vi "Core.vi"(8 "Mirrors& Splitters":map{cluster{i32, i32}, string}(c390), 9 "ySize":i32, 10 "xSize":i32, 11 "Initial Lazer":T1) -> (3 "Number Energized":i32)   [LabVIEW 2023, in "d16.lvlib"]
uses:
  d16.lvlib
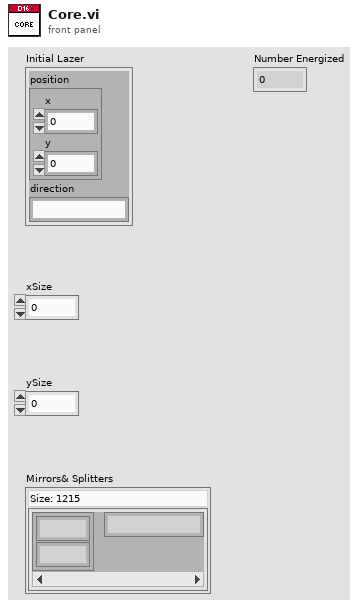
[diagram p1: front panel]
types:
  T1 = cluster{"position":cluster{"x":i32, "y":i32}, "direction":string}
  T2 = set{cluster{"position":cluster{"x":i32, "y":i32}, "direction":string}}
  T3 = cluster{"position":cluster{"x":i32, "y":i32}, "direction":string}[]
  T4 = cluster{"position":cluster{"x":i32, "y":i32}, string}
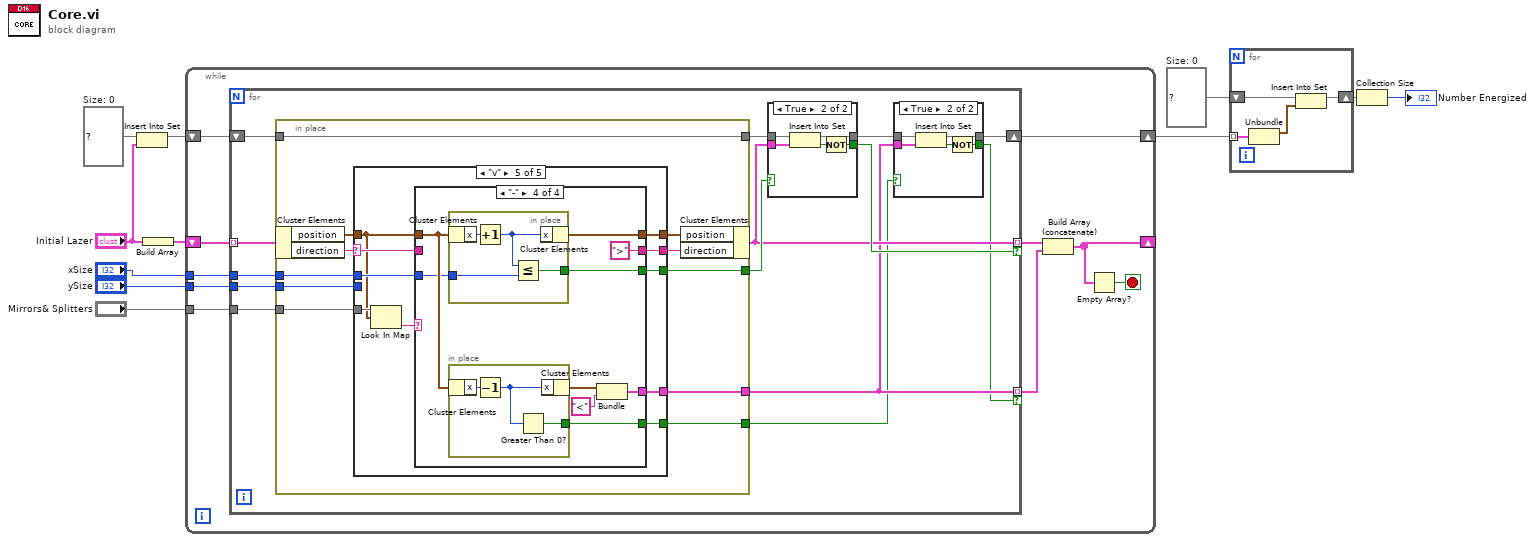
[diagram p0: block diagram]
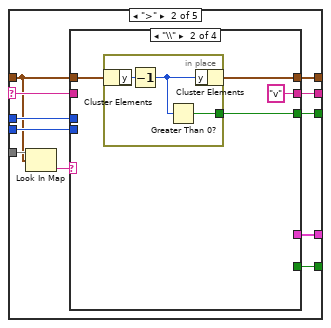
[diagram p5: hidden frame]
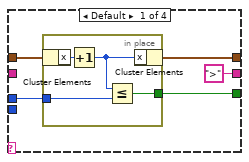
[diagram p6: hidden frame]
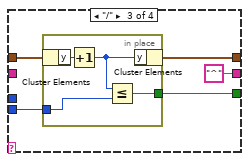
[diagram p7: hidden frame]
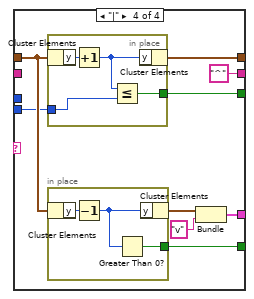
[diagram p8: hidden frame]
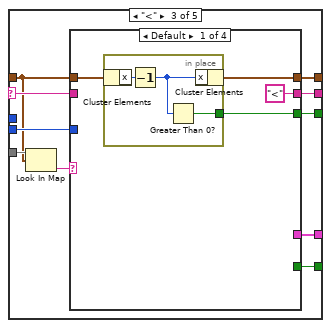
[diagram p9: hidden frame]
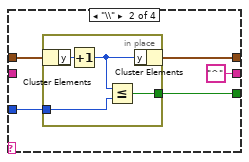
[diagram p10: hidden frame]
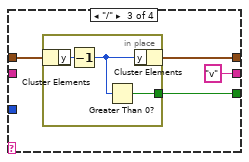
[diagram p11: hidden frame]
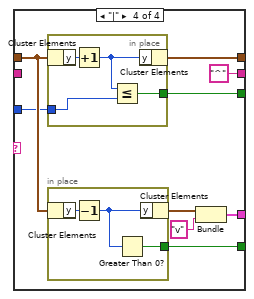
[diagram p12: hidden frame]
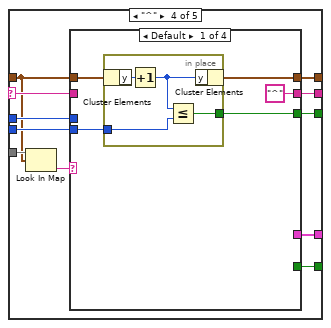
[diagram p13: hidden frame]
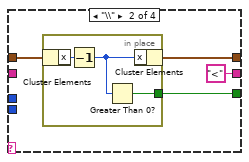
[diagram p14: hidden frame]
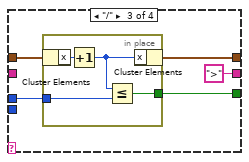
[diagram p15: hidden frame]
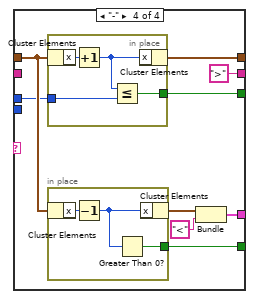
[diagram p16: hidden frame]
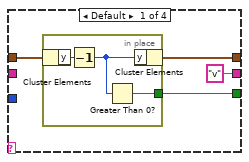
[diagram p17: hidden frame]
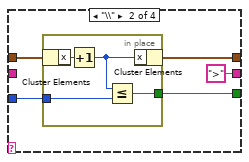
[diagram p18: hidden frame]
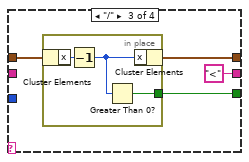
[diagram p19: hidden frame]
diagram:
  w10 = set{cluster{i32, i32}} {}  # Size: 0
  w6 = T2 {}  # Size: 0
  n1 = Insert Into Set(10:"Initial Lazer", 11:w6) -> (3:w7:T2)  [unwired: 1 out]
  n2 = Build Array("Initial Lazer") -> (w5:T3)
  n3 = while {
    tunnel: "xSize" -> [w17]
    tunnel: "ySize" -> [w14]
    shift-right: [w13] -> _
    shift-left: w5 -> [w19]
    tunnel: "Mirrors& Splitters" -> [w18]
    shift-right: [w20] -> w9
    shift-left: w7 -> [w21]
    stop <- w15 stop-if-true
    n4 = for {
      tunnel: w19 -> [w32] mode=indexing
      tunnel: w18 -> [w34]
      tunnel: w17 -> [w33]
      tunnel: [w27] -> w16 mode=indexing if=w28
      tunnel: w14 -> [w31]
      tunnel: [w24] -> w12 mode=indexing if=w22
      shift-right: [w25] -> w20
      shift-left: w21 -> [w35]
      n5 = in-place {
        in-place-border: w35 -> [w58]
        in-place-border: [w58] -> w30
        in-place-border: w34 -> [w57]
        in-place-border: w33 -> [w56]
        in-place-border: [w55] -> w29
        in-place-border: w31 -> [w50]
        in-place-border: [w49] -> w24
        in-place-border: [w48] -> w23
        n6 = in-place-cluster #1(w32) -> ("position"=w54:cluster{"x":i32, "y":i32}, "direction"=w51:string)
        n7 = case shown="\"v\"" w51 {
          selector: w51 -> [_ w65 w116 w166 w217]
          tunnel: w54 -> [w59 w60 w112 w161 w213]
          tunnel: w57 -> [_ w70 w121 w171 w222]
          tunnel: w56 -> [_ w64 _ w165 w216]
          tunnel: [_ w62 w114 w163 w214] -> w55
          tunnel: [_ w68 w119 w169 w220] -> w52
          tunnel: [w59 w63 w115 w164 w215] -> w53
          tunnel: w50 -> [_ w61 w113 w162 _]
          tunnel: [_ w67 w118 w168 w219] -> w48
          tunnel: [_ w66 w117 w167 w218] -> w49
          frame "False", Default {
          }
          frame ">" {
            n8 = Look In Map(map=w70, key=w60) -> (value=w69:string)  [unwired: 1 in, 1 out]
            n9 = case shown="\"\\\\\"" w69 {
              tunnel: [">" "v" "^" "^"] -> w68
              tunnel: [_ _ _ w96] -> w67
              tunnel: [_ _ _ w102] -> w66
              tunnel: w65 -> [_ _ _ _]
              tunnel: w60 -> [w75 w82 w90 w99]
              tunnel: w64 -> [w73 _ _ _]
              tunnel: [w74 w81 w89 w100] -> w63
              tunnel: [w72 w80 w87 w101] -> w62
              tunnel: w61 -> [_ _ w88 w98]
              frame Default {
                n10 = in-place {
                  in-place-border: [w78] -> w72
                  in-place-border: w73 -> [w76]
                  n11 = in-place-cluster #2(w75) -> ("x"=w79:i32)
                  n12 = Increment(x=w79) -> (x+1=w77:i32)
                  n13 = Less Or Equal?(x=w77, y=w76) -> (x <= y?=w78:bool)
                  n14 = in-place-cluster #2("x"=w77) -> (w74:cluster{"x":i32, "y":i32})
                }
              }
              frame "\\" {
                n15 = in-place {
                  in-place-border: [w85] -> w80
                  n16 = in-place-cluster #3(w82) -> ("y"=w86:i32)
                  n17 = Decrement(x=w86) -> (x-1=w84:i32)
                  n18 = Greater Than 0?(x=w84) -> (x > 0?=w85:bool)
                  n19 = in-place-cluster #3("y"=w84) -> (w81:cluster{"x":i32, "y":i32})
                }
              }
              frame "/" {
                n20 = in-place {
                  in-place-border: [w94] -> w87
                  in-place-border: w88 -> [w92]
                  n21 = in-place-cluster #4(w90) -> ("y"=w95:i32)
                  n22 = Increment(x=w95) -> (x+1=w93:i32)
                  n23 = Less Or Equal?(x=w93, y=w92) -> (x <= y?=w94:bool)
                  n24 = in-place-cluster #4("y"=w93) -> (w89:cluster{"x":i32, "y":i32})
                }
              }
              frame "|" {
                n25 = in-place {
                  in-place-border: [w107] -> w101
                  in-place-border: w98 -> [w105]
                  n26 = in-place-cluster #5(w99) -> ("y"=w108:i32)
                  n27 = Increment(x=w108) -> (x+1=w106:i32)
                  n28 = Less Or Equal?(x=w106, y=w105) -> (x <= y?=w107:bool)
                  n29 = in-place-cluster #5("y"=w106) -> (w100:cluster{"x":i32, "y":i32})
                }
                n30 = in-place {
                  in-place-border: [w109] -> w96
                  n31 = in-place-cluster #6(w99) -> ("y"=w111:i32)
                  n32 = Decrement(x=w111) -> (x-1=w110:i32)
                  n33 = Greater Than 0?(x=w110) -> (x > 0?=w109:bool)
                  n34 = in-place-cluster #6("y"=w110) -> (w104:cluster{"x":i32, "y":i32})
                }
                n35 = Bundle("position"=w104, "v") -> (w102:T4)  [unwired: 1 in]
              }
            }
          }
          frame "<" {
            n36 = Look In Map(map=w121, key=w112) -> (value=w120:string)  [unwired: 1 in, 1 out]
            n37 = case shown="Default" w120 {
              tunnel: ["<" "^" "v" "^"] -> w119
              tunnel: [_ _ _ w145] -> w118
              tunnel: [_ _ _ w151] -> w117
              tunnel: w116 -> [_ _ _ _]
              tunnel: w112 -> [w125 w132 w140 w148]
              tunnel: [w124 w131 w139 w149] -> w115
              tunnel: [w123 w130 w138 w150] -> w114
              tunnel: w113 -> [_ w129 _ w147]
              frame Default {
                n38 = in-place {
                  in-place-border: [w127] -> w123
                  n39 = in-place-cluster #7(w125) -> ("x"=w128:i32)
                  n40 = Decrement(x=w128) -> (x-1=w126:i32)
                  n41 = Greater Than 0?(x=w126) -> (x > 0?=w127:bool)
                  n42 = in-place-cluster #7("x"=w126) -> (w124:cluster{"x":i32, "y":i32})
                }
              }
              frame "\\" {
                n43 = in-place {
                  in-place-border: [w136] -> w130
                  in-place-border: w129 -> [w134]
                  n44 = in-place-cluster #8(w132) -> ("y"=w137:i32)
                  n45 = Increment(x=w137) -> (x+1=w135:i32)
                  n46 = Less Or Equal?(x=w135, y=w134) -> (x <= y?=w136:bool)
                  n47 = in-place-cluster #8("y"=w135) -> (w131:cluster{"x":i32, "y":i32})
                }
              }
              frame "/" {
                n48 = in-place {
                  in-place-border: [w143] -> w138
                  n49 = in-place-cluster #9(w140) -> ("y"=w144:i32)
                  n50 = Decrement(x=w144) -> (x-1=w142:i32)
                  n51 = Greater Than 0?(x=w142) -> (x > 0?=w143:bool)
                  n52 = in-place-cluster #9("y"=w142) -> (w139:cluster{"x":i32, "y":i32})
                }
              }
              frame "|" {
                n53 = in-place {
                  in-place-border: [w156] -> w150
                  in-place-border: w147 -> [w154]
                  n54 = in-place-cluster #10(w148) -> ("y"=w157:i32)
                  n55 = Increment(x=w157) -> (x+1=w155:i32)
                  n56 = Less Or Equal?(x=w155, y=w154) -> (x <= y?=w156:bool)
                  n57 = in-place-cluster #10("y"=w155) -> (w149:cluster{"x":i32, "y":i32})
                }
                n58 = in-place {
                  in-place-border: [w158] -> w145
                  n59 = in-place-cluster #11(w148) -> ("y"=w160:i32)
                  n60 = Decrement(x=w160) -> (x-1=w159:i32)
                  n61 = Greater Than 0?(x=w159) -> (x > 0?=w158:bool)
                  n62 = in-place-cluster #11("y"=w159) -> (w153:cluster{"x":i32, "y":i32})
                }
                n63 = Bundle("position"=w153, "v") -> (w151:T4)  [unwired: 1 in]
              }
            }
          }
          frame "^" {
            n64 = Look In Map(map=w171, key=w161) -> (value=w170:string)  [unwired: 1 in, 1 out]
            n65 = case shown="Default" w170 {
              tunnel: ["^" "<" ">" ">"] -> w169
              tunnel: [_ _ _ w198] -> w168
              tunnel: [_ _ _ w203] -> w167
              tunnel: w166 -> [_ _ _ _]
              tunnel: w161 -> [w176 w183 w191 w200]
              tunnel: w165 -> [_ _ w188 w197]
              tunnel: [w175 w182 w190 w201] -> w164
              tunnel: [w174 w181 w189 w202] -> w163
              tunnel: w162 -> [w172 _ _ _]
              frame Default {
                n66 = in-place {
                  in-place-border: [w179] -> w174
                  in-place-border: w172 -> [w177]
                  n67 = in-place-cluster #12(w176) -> ("y"=w180:i32)
                  n68 = Increment(x=w180) -> (x+1=w178:i32)
                  n69 = Less Or Equal?(x=w178, y=w177) -> (x <= y?=w179:bool)
                  n70 = in-place-cluster #12("y"=w178) -> (w175:cluster{"x":i32, "y":i32})
                }
              }
              frame "\\" {
                n71 = in-place {
                  in-place-border: [w186] -> w181
                  n72 = in-place-cluster #13(w183) -> ("x"=w187:i32)
                  n73 = Decrement(x=w187) -> (x-1=w185:i32)
                  n74 = Greater Than 0?(x=w185) -> (x > 0?=w186:bool)
                  n75 = in-place-cluster #13("x"=w185) -> (w182:cluster{"x":i32, "y":i32})
                }
              }
              frame "/" {
                n76 = in-place {
                  in-place-border: [w195] -> w189
                  in-place-border: w188 -> [w193]
                  n77 = in-place-cluster #14(w191) -> ("x"=w196:i32)
                  n78 = Increment(x=w196) -> (x+1=w194:i32)
                  n79 = Less Or Equal?(x=w194, y=w193) -> (x <= y?=w195:bool)
                  n80 = in-place-cluster #14("x"=w194) -> (w190:cluster{"x":i32, "y":i32})
                }
              }
              frame "-" {
                n81 = in-place {
                  in-place-border: [w208] -> w202
                  in-place-border: w197 -> [w206]
                  n82 = in-place-cluster #15(w200) -> ("x"=w209:i32)
                  n83 = Increment(x=w209) -> (x+1=w207:i32)
                  n84 = Less Or Equal?(x=w207, y=w206) -> (x <= y?=w208:bool)
                  n85 = in-place-cluster #15("x"=w207) -> (w201:cluster{"x":i32, "y":i32})
                }
                n86 = in-place {
                  in-place-border: [w210] -> w198
                  n87 = in-place-cluster #16(w200) -> ("x"=w212:i32)
                  n88 = Decrement(x=w212) -> (x-1=w211:i32)
                  n89 = Greater Than 0?(x=w211) -> (x > 0?=w210:bool)
                  n90 = in-place-cluster #16("x"=w211) -> (w205:cluster{"x":i32, "y":i32})
                }
                n91 = Bundle("position"=w205, "<") -> (w203:T4)  [unwired: 1 in]
              }
            }
          }
          frame "v" {
            n92 = Look In Map(map=w222, key=w213) -> (value=w221:string)  [unwired: 1 in, 1 out]
            n93 = case shown="\"-\"" w221 {
              tunnel: ["v" ">" "<" ">"] -> w220
              tunnel: [_ _ _ w247] -> w219
              tunnel: [_ _ _ w252] -> w218
              tunnel: w217 -> [_ _ _ _]
              tunnel: w213 -> [w226 w233 w241 w249]
              tunnel: w216 -> [_ w230 _ w246]
              tunnel: [w225 w232 w240 w250] -> w215
              tunnel: [w224 w231 w239 w251] -> w214
              frame Default {
                n94 = in-place {
                  in-place-border: [w228] -> w224
                  n95 = in-place-cluster #17(w226) -> ("y"=w229:i32)
                  n96 = Decrement(x=w229) -> (x-1=w227:i32)
                  n97 = Greater Than 0?(x=w227) -> (x > 0?=w228:bool)
                  n98 = in-place-cluster #17("y"=w227) -> (w225:cluster{"x":i32, "y":i32})
                }
              }
              frame "\\" {
                n99 = in-place {
                  in-place-border: [w237] -> w231
                  in-place-border: w230 -> [w235]
                  n100 = in-place-cluster #18(w233) -> ("x"=w238:i32)
                  n101 = Increment(x=w238) -> (x+1=w236:i32)
                  n102 = Less Or Equal?(x=w236, y=w235) -> (x <= y?=w237:bool)
                  n103 = in-place-cluster #18("x"=w236) -> (w232:cluster{"x":i32, "y":i32})
                }
              }
              frame "/" {
                n104 = in-place {
                  in-place-border: [w244] -> w239
                  n105 = in-place-cluster #19(w241) -> ("x"=w245:i32)
                  n106 = Decrement(x=w245) -> (x-1=w243:i32)
                  n107 = Greater Than 0?(x=w243) -> (x > 0?=w244:bool)
                  n108 = in-place-cluster #19("x"=w243) -> (w240:cluster{"x":i32, "y":i32})
                }
              }
              frame "-" {
                n109 = in-place {
                  in-place-border: [w257] -> w251
                  in-place-border: w246 -> [w255]
                  n110 = in-place-cluster #20(w249) -> ("x"=w258:i32)
                  n111 = Increment(x=w258) -> (x+1=w256:i32)
                  n112 = Less Or Equal?(x=w256, y=w255) -> (x <= y?=w257:bool)
                  n113 = in-place-cluster #20("x"=w256) -> (w250:cluster{"x":i32, "y":i32})
                }
                n114 = in-place {
                  in-place-border: [w259] -> w247
                  n115 = in-place-cluster #21(w249) -> ("x"=w261:i32)
                  n116 = Decrement(x=w261) -> (x-1=w260:i32)
                  n117 = Greater Than 0?(x=w260) -> (x > 0?=w259:bool)
                  n118 = in-place-cluster #21("x"=w260) -> (w254:cluster{"x":i32, "y":i32})
                }
                n119 = Bundle("position"=w254, "<") -> (w252:T4)  [unwired: 1 in]
              }
            }
          }
        }
        n120 = in-place-cluster #1("position"=w53, "direction"=w52) -> (w27:T1)
      }
      n121 = case shown="True" w29 {
        tunnel: w30 -> [w42 w47]
        tunnel: [_ w44] -> w28
        tunnel: w27 -> [_ w45]
        tunnel: [w42 w43] -> w26
        frame False {
        }
        frame True {
          n122 = Insert Into Set(10:w45, 11:w47) -> (2:w46:bool, 3:w43:T2)
          n123 = Not(x=w46) -> (.not. x?=w44:bool)
        }
      }
      n124 = case shown="True" w23 {
        tunnel: w26 -> [w36 w41]
        tunnel: [_ w38] -> w22
        tunnel: w24 -> [_ w39]
        tunnel: [w36 w37] -> w25
        frame False {
        }
        frame True {
          n125 = Insert Into Set(10:w39, 11:w41) -> (2:w40:bool, 3:w37:T2)
          n126 = Not(x=w40) -> (.not. x?=w38:bool)
        }
      }
    }
    n127 = Build Array (concatenate)(w16, w12) -> (w13:T3)
    n128 = Empty Array?(array=w13) -> (empty?=w15:bool)
  }
  n129 = for {
    tunnel: w9 -> [w263] mode=indexing
    shift-right: [w264] -> w11
    shift-left: w10 -> [w265]
    n130 = Unbundle(w263) -> ("position"=w262:cluster{"x":i32, "y":i32})  [unwired: 1 out]
    n131 = Insert Into Set(10:w262, 11:w265) -> (3:w264:set{cluster{i32, i32}})  [unwired: 1 out]
  }
  n132 = Collection Size(1:w11) -> (0:→"Number Energized":i32)
